vi "Read WriteUrgent.vi"(8 "error in (no error)":errorcluster, 11 "WebSocket Data Model in":refnum<class "WebSocket Data Model.lvclass">) -> (0 "error out":errorcluster, 2 "WriteUrgent":refnum<user-event>, 3 "WebSocket Data Model out":refnum<class "WebSocket Data Model.lvclass">)   [LabVIEW 2021, in "WebSockets.lvlib" / "WebSocket Data Model.lvclass"]
uses:
  WebSocket Data Model.lvclass
  WebSocket/Opcodes.ctl
  WebSocket Data Model.lvclass/WebSocket Data Model.ctl
  WebSocket/WebSocket.lvclass
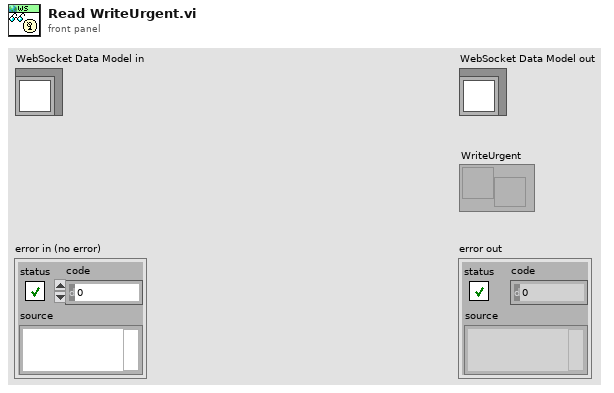
[diagram p1: front panel]
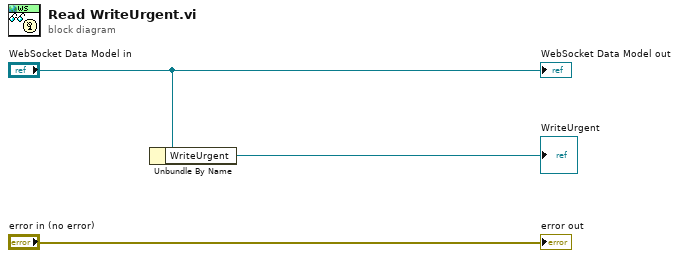
[diagram p0: block diagram]
diagram:
  n1 = Unbundle By Name("WebSocket Data Model in") -> ("WriteUrgent"=→"WriteUrgent":refnum<user-event>)
  "error out" <- "error in (no error)"
  "WebSocket Data Model out" <- "WebSocket Data Model in"
